vi "1.1.vi"() -> ()   [LabVIEW 2020]
panel:
  out "Boolean 14":bool
  out "Boolean 13":bool
  out "Boolean 12":bool
  out "Boolean 11":bool
  out "Boolean 10":bool
  out "Boolean 9":bool
  out "Boolean 8":bool
  in  "Boolean 7":bool
  in  "Boolean 6":bool
  in  "Boolean 5":bool
  in  "Boolean 4":bool
  in  "Boolean 3":bool
  in  "Boolean 2":bool
  in  "Boolean":bool
  # "Enciendte esto ->"
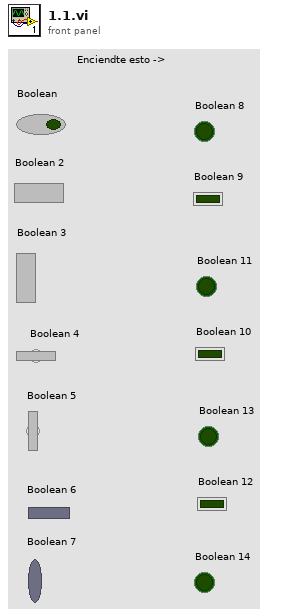
[diagram p1: front panel]
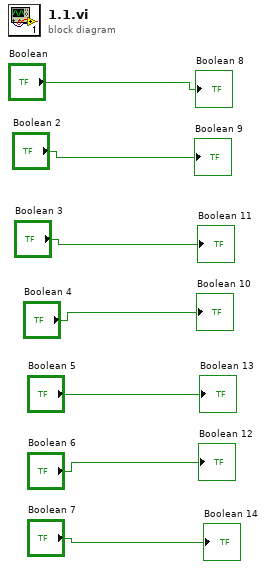
[diagram p0: block diagram]
diagram:
  "Boolean 8" <- "Boolean"
  "Boolean 9" <- "Boolean 2"
  "Boolean 11" <- "Boolean 3"
  "Boolean 10" <- "Boolean 4"
  "Boolean 13" <- "Boolean 5"
  "Boolean 12" <- "Boolean 6"
  "Boolean 14" <- "Boolean 7"
